vi "ConfMaker.vi"() -> ()   [LabVIEW 2012]
uses:
  <vilib>/Utility/config.llb/Write Key (String).vi
  <vilib>/Utility/config.llb/NI_LVConfig.lvlib
panel:
  in  "Path":path
  in  "Sections":string[][][](array[string])
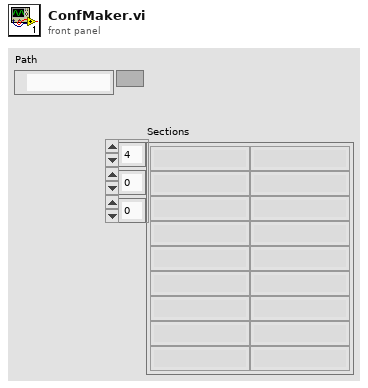
[diagram p1: front panel]
types:
  T1 = typedef "NI_LVConfig.lvlib/Config Data RefNum.ctl" = refnum<k1>
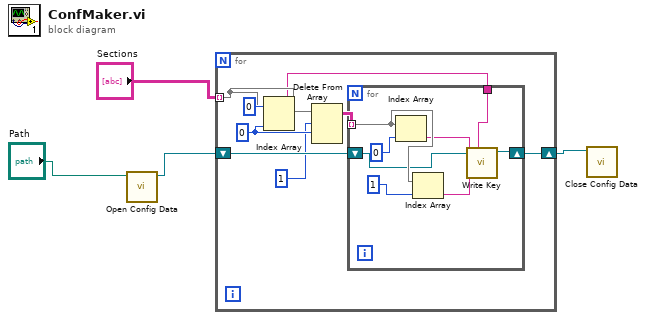
[diagram p0: block diagram]
diagram:
  n1 = call <vilib>:"Open Config Data.vi"("configuration file path"="Path") -> ("refnum"=w3:T1)  [unwired: 8 in, 2 out]
  n2 = for {
    tunnel: "Sections" -> [w11] mode=indexing
    shift-right: [w6] -> w2
    shift-left: w3 -> [w7]
    w9 = 0
    n3 = Index Array(array=w11, index (row)=0, index (col)=w9) -> (element=w8:string)
    n4 = Delete From Array(array=w11, length=1, index (row)=w9) -> (array with subset deleted=w10:string[][])  [unwired: 1 in, 1 out]
    n5 = for {
      tunnel: w10 -> [w18] mode=indexing
      tunnel: w8 -> [w17]
      shift-right: [w14] -> w6
      shift-left: w7 -> [w13]
      n6 = Index Array(array=w18, index=0) -> (element=w16:string)
      n7 = Index Array(array=w18, index=1) -> (element=w15:string)
      n8 = call-poly <vilib>:"Write Key.vi"("section"=w17, "value"=w15, "key"=w16, "refnum"=w13) -> ("refnum out"=w14:T1)  [unwired: 5 in, 2 out]
    }
  }
  n9 = call <vilib>:"Close Config Data.vi"("refnum"=w2) -> ()  [unwired: 9 in, 2 out]
